vi "Configure Temperature.vi"   [LabVIEW 2013, in "Keithley 27XX.lvlib"]
doc: "This VI is used to configure the various settings for temperature measurements. It will set the transducer type to the polymorphic case selected."
uses:
  <instrlib>/Keithley 27XX/Keithley 27XX.lvlib
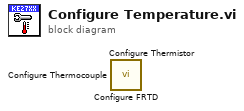
[diagram p0: block diagram]
diagram:
  n1 = call <instrlib>:"Configure FRTD.vi"() -> ()  [unwired: 18 in, 2 out]
  n2 = call <instrlib>:"Configure Thermistor.vi"() -> ()  [unwired: 18 in, 2 out]
  n3 = call <instrlib>:"Configure Thermocouple.vi"() -> ()  [unwired: 18 in, 2 out]
